vi "use_or_discard_data.vi"(1 "Status":string) -> (0 "use data":bool)   [LabVIEW 2018]
panel:
  # "832\n1101000000"
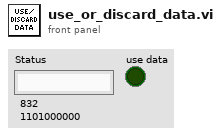
[diagram p1: front panel]
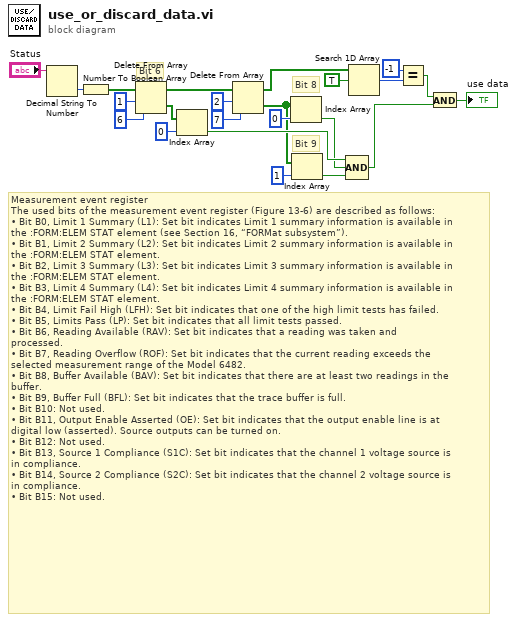
[diagram p0: block diagram]
diagram:
  # "Measurement event register\nThe used bits of the measurement event register (Figure 13-6) are described as follows:\n• Bit B0, Limit 1 Summary (L1): Set bit indicates Limit 1 summary information is available in\nthe :FORM:ELEM STAT element (see Section 16, “FORMat subsystem”).\n• Bit B1, Limit 2 Summary (L2): Set bit indicates Limit 2 summary information is available in\nthe :FORM:ELEM STAT element.\n• Bit B2, Limit 3 Summary (L3): Set bit indicates Limit 3 summary information is available in\nthe :FORM:ELEM STAT element.\n• Bit B3, Limit 4 Summary (L4): Set bit indicates Limit 4 summary information is available in\nthe :FORM:ELEM STAT element.\n• Bit B4, Limit Fail High (LFH): Set bit indicates that one of the high limit tests has failed.\n• Bit B5, Limits Pass (LP): Set bit indicates that all limit tests passed.\n• Bit B6, Reading Available (RAV): Set bit indicates that a reading was taken and\nprocessed.\n• Bit B7, Reading Overflow (ROF): Set bit indicates that the current reading exceeds the\nselected measurement range of the Model 6482.\n• Bit B8, Buffer Available (BAV): Set bit indicates that there are at least two readings in the\nbuffer.\n• Bit B9, Buffer Full (BFL): Set bit indicates that the trace buffer is full.\n• Bit B10: Not used.\n• Bit B11, Output Enable Asserted (OE): Set bit indicates that the output enable line is at\ndigital low (asserted). Source outputs can be turned on.\n• Bit B12: Not used.\n• Bit B13, Source 1 Compliance (S1C): Set bit indicates that the channel 1 voltage source is\nin compliance.\n• Bit B14, Source 2 Compliance (S2C): Set bit indicates that the channel 2 voltage source is\nin compliance.\n• Bit B15: Not used."
  # "Bit 9"
  # "Bit 8"
  # "Bit 6"
  n1 = Decimal String To Number(string="Status") -> (number=w2:i32)  [unwired: 3 out]
  n2 = Number To Boolean Array(number=w2) -> (Boolean array=w23:bool[])
  n3 = Delete From Array(array=w23, length=1, index=6) -> (deleted portion=w17:bool[], array with subset deleted=w18:bool[])
  n4 = Index Array(array=w17, index=0) -> (element=w16:bool)
  n5 = Delete From Array(array=w18, length=2, index=7) -> (deleted portion=w12:bool[], array with subset deleted=w8:bool[])
  n6 = Index Array(array=w12, index=0) -> (element=w11:bool)
  n7 = Index Array(array=w12, index=1) -> (element=w10:bool)
  n8 = Compound Arithmetic op=AND(w16, w11, w10) -> (w9:bool)
  n9 = Search 1D Array(1D array=w8, element=TRUE) -> (index of element=w5:i32)  [unwired: 1 in]
  n10 = Equal?(x=-1, y=w5) -> (x = y?=w3:bool)
  n11 = And(x=w3, y=w9) -> (x .and. y?=→"use data":bool)
